vi "Open Event Filter Reference.vi"(8 "error in (no error)":errorcluster, 11 "IEventFilter in":refnum<class "IEventFilter.lvclass">) -> (0 "error out":errorcluster, 3 "IEventFilter Reference":T1)   [LabVIEW 2019, in "ActorEvents.lvlib" / "IEventFilter.lvclass"]
uses:
  <vilib>/gpm_packages/@cs/mva-viewable/Source/ActorEvents/IEventFilter/IEventFilter.lvclass
  <vilib>/gpm_packages/@cs/mva-viewable/Source/ActorEvents/IEventFilter/EventFilter Reference.ctl
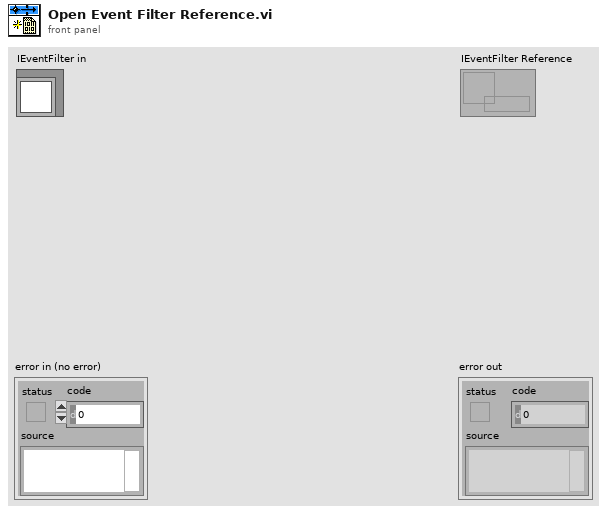
[diagram p1: front panel]
types:
  T1 = typedef "ActorEvents.lvlib/IEventFilter.lvclass/EventFilter Reference.ctl" = refnum<data-value>
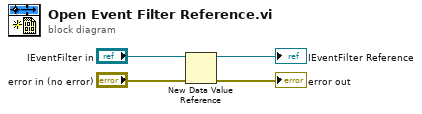
[diagram p0: block diagram]
diagram:
  n1 = New Data Value Reference(data value="IEventFilter in", error in="error in (no error)") -> (data value reference=→"IEventFilter Reference":refnum<data-value>, error out=→"error out":errorcluster)
